vi "Write Medio Comunicacion.vi"(8 "error in (no error)":errorcluster, 10 "Medio Comunicacion":string, 11 "Instrumento in":refnum<class "Instrumento.lvclass">) -> (0 "error out":errorcluster, 3 "Instrumento out":refnum<class "Instrumento.lvclass">)   [LabVIEW 2020, in "Instrumento.lvclass"]
uses:
  Instrumento.lvclass
  Instrumento.lvclass/Instrumento.ctl
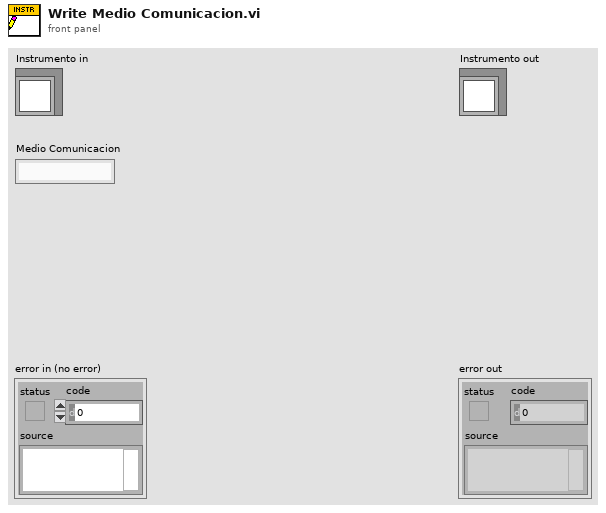
[diagram p1: front panel]
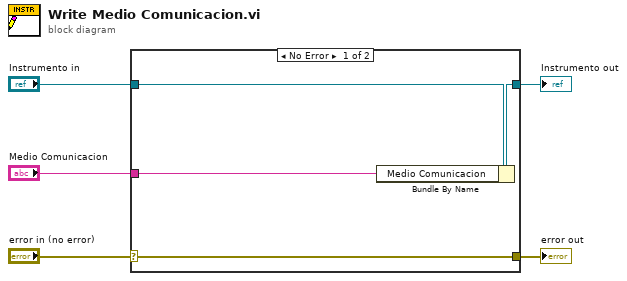
[diagram p0: block diagram]
diagram:
  n1 = case shown="No Error" "error in (no error)" {
    selector: "error in (no error)" -> [w9 w10]
    tunnel: [w9 w10] -> w4
    tunnel: [w7 w11] -> w2
    tunnel: "Instrumento in" -> [w8 w11]
    tunnel: "Medio Comunicacion" -> [w6 _]
    frame No Error {
      n2 = Bundle By Name(cluster=w8, "Medio Comunicacion"=w6) -> (w7:refnum<class "Instrumento.lvclass">)
    }
    frame Error {
    }
  }
  "error out" <- w4
  "Instrumento out" <- w2
